vi "FGV.vi"(0 "Serial Device in":refnum<class "Serial Device.lvclass">, 1 "Enum":enum16{"Get Data", "Set Data"}(ring), 2 "Name":string, 3 "error in (no error)":errorcluster, 4 "Data 2":variant) -> (7 "Serial Device out":refnum<class "Serial Device.lvclass">, 9 "Data":variant, 10 "error out":errorcluster)   [LabVIEW 2020, in "Serial Device.lvclass"]
uses:
  Serial Device.lvclass
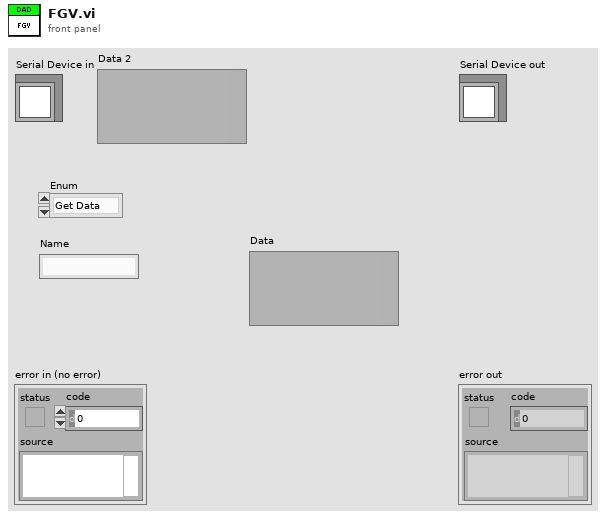
[diagram p1: front panel]
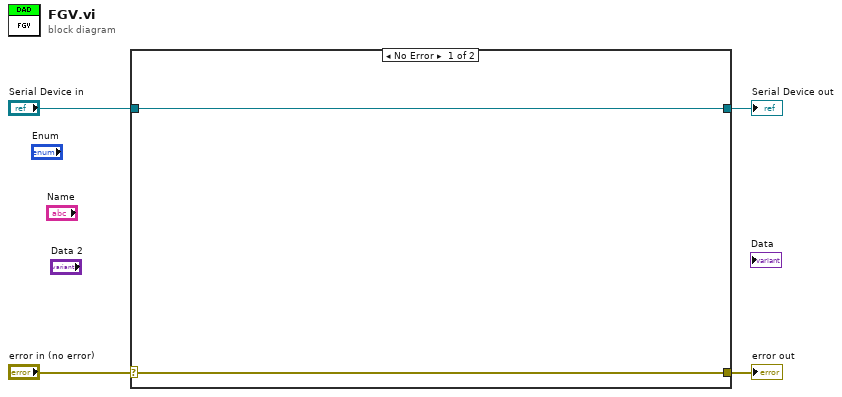
[diagram p0: block diagram]
diagram:
  n1 = case shown="No Error" "error in (no error)" {
    selector: "error in (no error)" -> [w5 w8]
    tunnel: [w5 w8] -> w3
    tunnel: [w6 w7] -> w1
    tunnel: "Serial Device in" -> [w6 w7]
    frame No Error {
    }
    frame Error {
    }
  }
  "error out" <- w3
  "Serial Device out" <- w1
